vi "Calculate.vi"(7 "Conversion":refnum<k21>, 8 "error in (no error)":errorcluster, 9 "PCL dt":dbl, 10 "Values":dbl[](array[numeric]), 11 "Frame Configuration":T1 {"CRC"."Data Type" items=["Signed", "Unsigned", "IEEE Float"]; "Rolling Counter"."Data Type" items=["Signed", "Unsigned", "IEEE Float"]; "Input Channels"."Data Type" items=["Signed", "Unsigned", "IEEE Float"]}) -> (0 "error out":errorcluster, 1 "ProtectionValue":dbl, 2 "Rolling Counter":dbl, 3 "Frame Configuration":T1 {"CRC"."Data Type" items=["Signed", "Unsigned", "IEEE Float"]; "Rolling Counter"."Data Type" items=["Signed", "Unsigned", "IEEE Float"]; "Input Channels"."Data Type" items=["Signed", "Unsigned", "IEEE Float"]})   [LabVIEW 2016, in "LIN Frame Protection Addon Engine.lvlib"]
uses:
  LIN Frame Protection Addon Engine.lvlib
  Shared/Types/FrameConfiguration.ctl
  Shared/Types/InputChannelConfiguration.ctl
  Shared/Types/Protection Type.ctl
  <vilib>/xnet/xnet.llb/XNET Convert (Signal to Frame Raw).vi
  Shared/LIN Frame Protection Addon Shared.lvlib
panel:
  out "PCLIterations":dbl
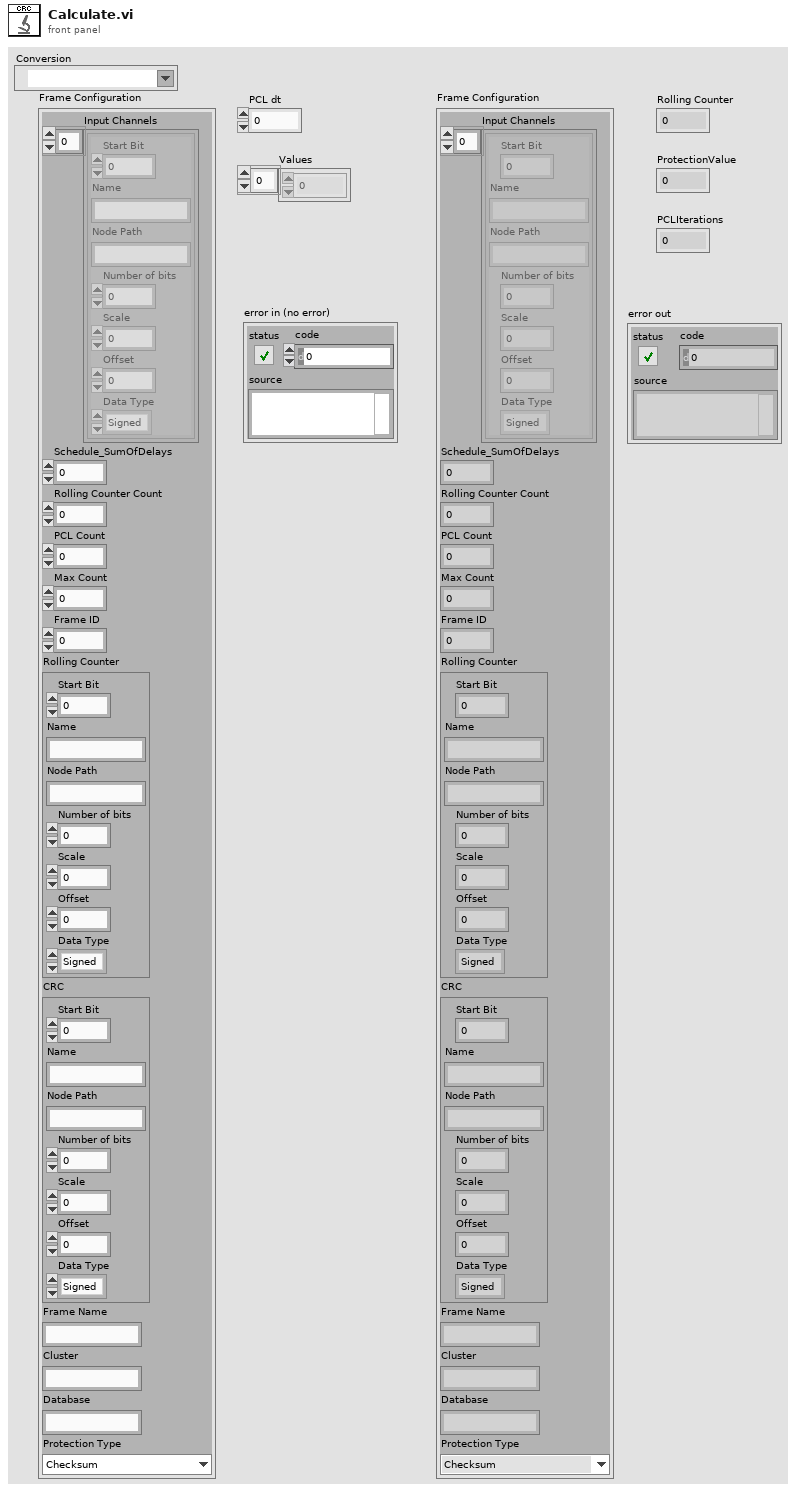
[diagram p1: front panel]
types:
  T1 = typedef "LIN Frame Protection Addon Shared.lvlib/FrameConfiguration.ctl" = cluster{"Input Channels":T2[], "Schedule_SumOfDelays":dbl, "Rolling Counter Count":dbl, "PCL Count":u64, "Max Count":dbl, "Frame ID":u32, "Rolling Counter":T2, "CRC":T2, "Frame Name":string, "Cluster":string, "Database":string, "Protection Type":T3}
  T2 = typedef "LIN Frame Protection Addon Shared.lvlib/InputChannelConfiguration.ctl" = cluster{"Start Bit":i32, "Name":string, "Node Path":string, "Number of bits":i32, "Scale":dbl, "Offset":dbl, "Data Type":u32}
  T3 = typedef "LIN Frame Protection Addon Shared.lvlib/Protection Type.ctl" = enum16{"Checksum", "CRC", "None (Counter Only)"}
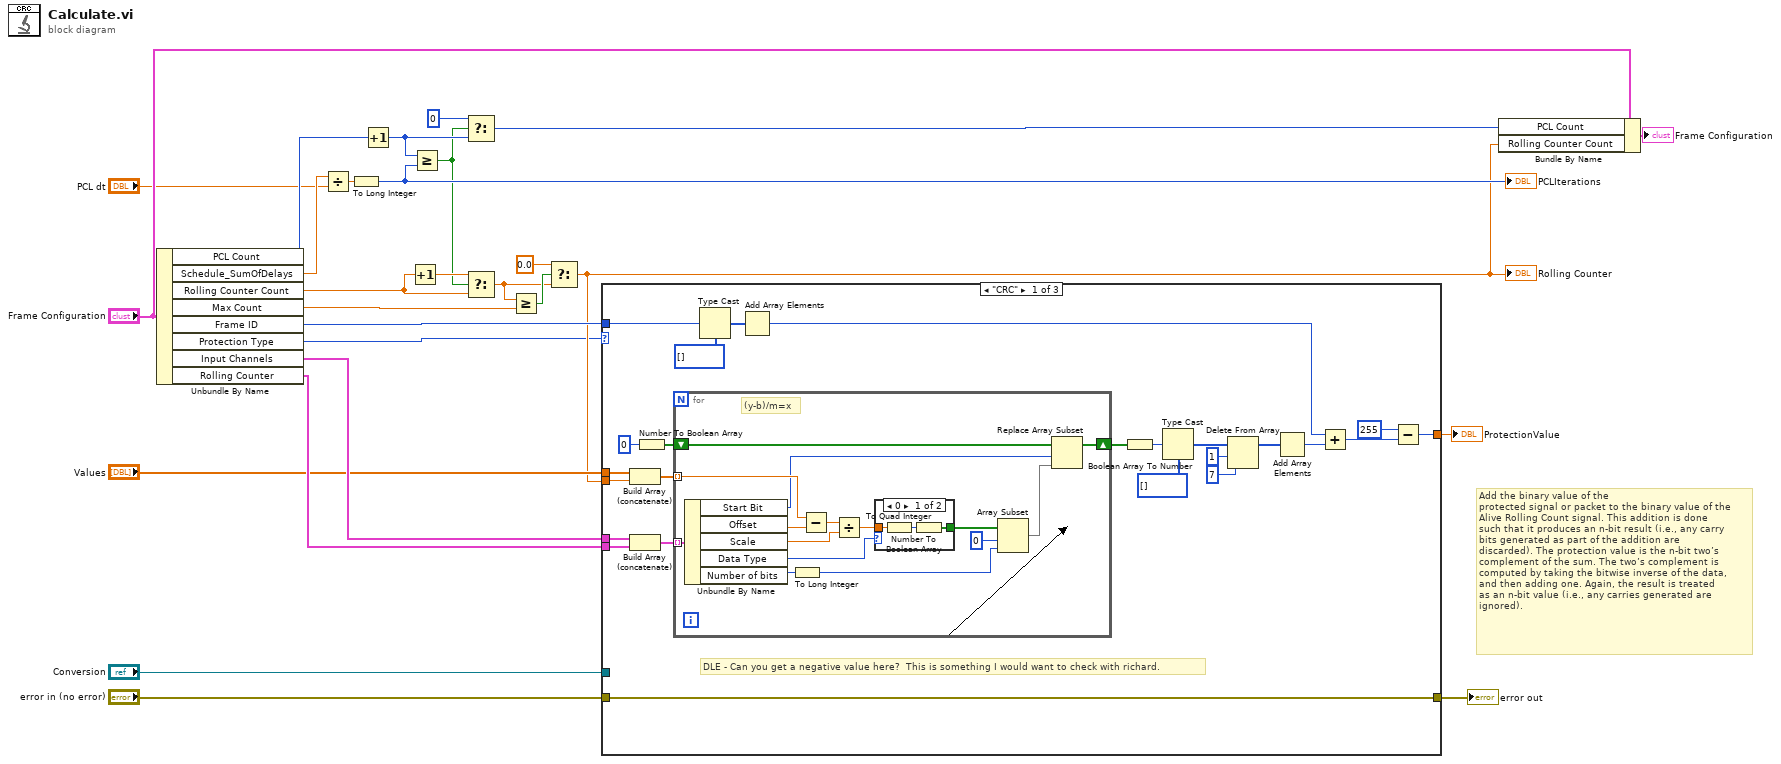
[diagram p0: block diagram]
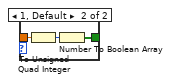
[diagram p2: hidden frame]
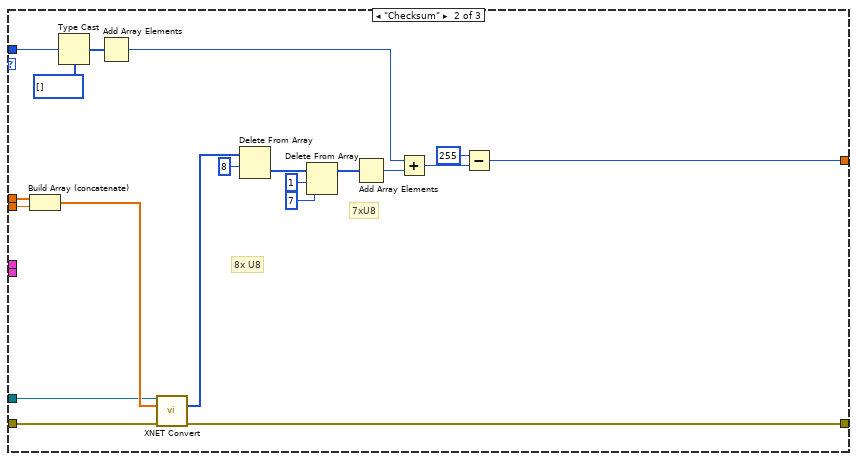
[diagram p3: hidden frame]
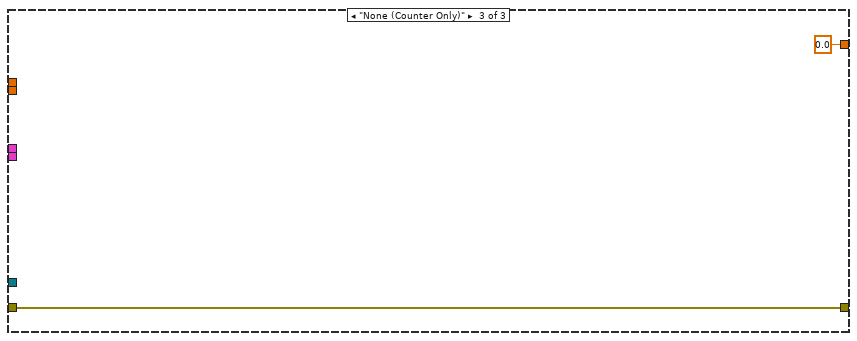
[diagram p4: hidden frame]
diagram:
  # "Add the binary value of the\nprotected signal or packet to the binary value of the\nAlive Rolling Count signal. This addition is done\nsuch that it produces an n-bit result (i.e., any carry\nbits generated as part of the addition are\ndiscarded). The protection value is the n-bit two’s\ncomplement of the sum. The two’s complement is\ncomputed by taking the bitwise inverse of the data,\nand then adding one. Again, the result is treated\nas an n-bit value (i.e., any carries generated are\nignored)."
  n1 = Unbundle By Name("Frame Configuration") -> ("PCL Count"=w22:u64, "Schedule_SumOfDelays"=w19:dbl, "Rolling Counter Count"=w20:dbl, "Max Count"=w16:dbl, "Frame ID"=w10:u32, "Protection Type"=w1:T3, "Input Channels"=w8:T2[], "Rolling Counter"=w7:T2)
  n2 = Divide(x=w19, y="PCL dt") -> (x/y=w27:dbl)
  n3 = To Long Integer(number=w27) -> (32bit integer=w15:i32)
  "PCLIterations" <- w15
  n4 = Increment(x=w22) -> (x+1=w14:u64)
  n5 = Increment(x=w20) -> (x+1=w26:dbl)
  n6 = Greater Or Equal?(x=w14, y=w15) -> (x >= y?=w11:bool)
  n7 = Select(t=u64 0, s=w11, f=w14) -> (s? t:f=w12:u64)
  n8 = Select(t=w26, s=w11, f=w20) -> (s? t:f=w24:dbl)
  n9 = Greater Or Equal?(x=w24, y=w16) -> (x >= y?=w25:bool)
  n10 = Select(t=0.0, s=w25, f=w24) -> (s? t:f=w5:dbl)
  "Rolling Counter" <- w5
  n11 = case shown="\"CRC\"" w1 {
    tunnel: w10 -> [w45 w86 _]
    tunnel: [w40 w81 0.0] -> w9
    tunnel: w8 -> [w39 _ _]
    tunnel: w7 -> [w38 _ _]
    tunnel: "Values" -> [w37 w80 _]
    tunnel: w5 -> [w36 w79 _]
    tunnel: "error in (no error)" -> [w28 w77 w94]
    tunnel: [w28 w76 w94] -> w3
    tunnel: "Conversion" -> [_ w75 _]
    frame "CRC" {
      # "DLE - Can you get a negative value here?  This is something I would want to check with richard."
      n12 = Build Array (concatenate)(w37, w36) -> (w35:dbl[])
      n13 = Build Array (concatenate)(w39, w38) -> (w29:T2[])
      n14 = Number To Boolean Array(number=u64 0) -> (Boolean array=w34:bool[])
      n15 = for {
        tunnel: w29 -> [w66] mode=indexing
        shift-right: [w57] -> w32
        shift-left: w34 -> [w59]
        tunnel: w35 -> [w56] mode=indexing
        # "(y-b)/m=x"
        n16 = Unbundle By Name(w66) -> ("Start Bit"=w53:i32, "Offset"=w65:dbl, "Scale"=w63:dbl, "Data Type"=w55:u32, "Number of bits"=w61:i32)
        n17 = To Long Integer(number=w61) -> (32bit integer=w52:i32)
        n18 = Subtract(x=w56, y=w65) -> (x-y=w64:dbl)
        n19 = Divide(x=w64, y=w63) -> (x/y=w62:dbl)
        n20 = case shown="0" w55 {
          tunnel: w62 -> [w69 w72]
          tunnel: [w67 w70] -> w54
          frame 0 {
            n21 = To Quad Integer(1:w69) -> (0:w68:i64)
            n22 = Number To Boolean Array(number=w68) -> (Boolean array=w67:bool[])
          }
          frame 1, Default {
            n23 = To Unsigned Quad Integer(1:w72) -> (0:w71:u64)
            n24 = Number To Boolean Array(number=w71) -> (Boolean array=w70:bool[])
          }
        }
        n25 = Array Subset(array=w54, index=0, length=w52) -> (w58:bool[])
        n26 = Replace Array Subset(array=w59, new element=w58, index=w53) -> (w57:bool[])
      }
      n27 = Type Cast(type=u8[] [], x=w45) -> (*(type *) &x=w44:u8[])
      n28 = Add Array Elements(numeric array=w44) -> (sum=w43:u8)
      n29 = Boolean Array To Number(Boolean array=w32) -> (number=w31:u64)
      n30 = Type Cast(type=u8[] [], x=w31) -> (*(type *) &x=w51:u8[])
      n31 = Delete From Array(array=w51, length=1, index=7) -> (array with subset deleted=w48:u8[])  [unwired: 1 out]
      n32 = Add Array Elements(numeric array=w48) -> (sum=w47:u8)
      n33 = Add(x=w43, y=w47) -> (x+y=w42:u8)
      n34 = Subtract(x=u8 255, y=w42) -> (x-y=w40:u8)
    }
    frame "Checksum" {
      # "7xU8"
      # "8x U8"
      n35 = Build Array (concatenate)(w80, w79) -> (w78:dbl[])
      n36 = Type Cast(type=u8[] [], x=w86) -> (*(type *) &x=w85:u8[])
      n37 = Add Array Elements(numeric array=w85) -> (sum=w84:u8)
      n38 = call-poly <vilib>:"XNET Convert.vi"("session in"=w75, "signal data"=w78, "error in (no error)"=w77) -> ("frame data"=w73:u8[], "error out"=w76:errorcluster)  [unwired: 10 in, 1 out]
      n39 = Delete From Array(array=w73, length=8) -> (deleted portion=w92:u8[])  [unwired: 1 in, 1 out]
      n40 = Delete From Array(array=w92, length=1, index=7) -> (array with subset deleted=w89:u8[])  [unwired: 1 out]
      n41 = Add Array Elements(numeric array=w89) -> (sum=w88:u8)
      n42 = Add(x=w84, y=w88) -> (x+y=w83:u8)
      n43 = Subtract(x=u8 255, y=w83) -> (x-y=w81:u8)
    }
    frame "None (Counter Only)" {
    }
  }
  "ProtectionValue" <- w9
  "error out" <- w3
  n44 = Bundle By Name(cluster="Frame Configuration", "PCL Count"=w12, "Rolling Counter Count"=w5) -> (→"Frame Configuration":T1)
